vi "Calc Texel Starting Conditions.vi"(10 "Texture":T5, 11 "Sorted Triangle":T1={"Top Vertex"={"Position"={"x"=0.0, "y"=0.0, "z"=0.0}, "UV"={"u"=0.0, "v"=0.0}, "Colour"=12517256}, "Mid Vertex"={"Position"={"x"=0.0, "y"=0.0, "z"=0.0}, "UV"={"u"=0.0, "v"=0.0}, "Colour"=12517256}, "Bottom Vertex"={"Position"={"x"=0.0, "y"=0.0, "z"=0.0}, "UV"={"u"=0.0, "v"=0.0}, "Colour"=12517256}, "Colour"=0} {"Bottom Vertex"."UV"."v" min=0 max=1 step=0.1; "Bottom Vertex"."UV"."u" min=0 max=1 step=0.1; "Mid Vertex"."UV"."v" min=0 max=1 step=0.1; "Mid Vertex"."UV"."u" min=0 max=1 step=0.1; "Top Vertex"."UV"."v" min=0 max=1 step=0.1; "Top Vertex"."UV"."u" min=0 max=1 step=0.1}) -> (3 "Step Deltas (Texels Per Step)":T7)   [LabVIEW 2020]
uses:
  Texel Step Deltas.ctl
  Raster (FPGA).lvlib
  Point 2D (SGL).ctl
  UV.ctl
  Rectangle Dimensions.ctl
  Texture.ctl
  Vector 3D.ctl
  Vertex.ctl
  Triangle (Sorted).ctl
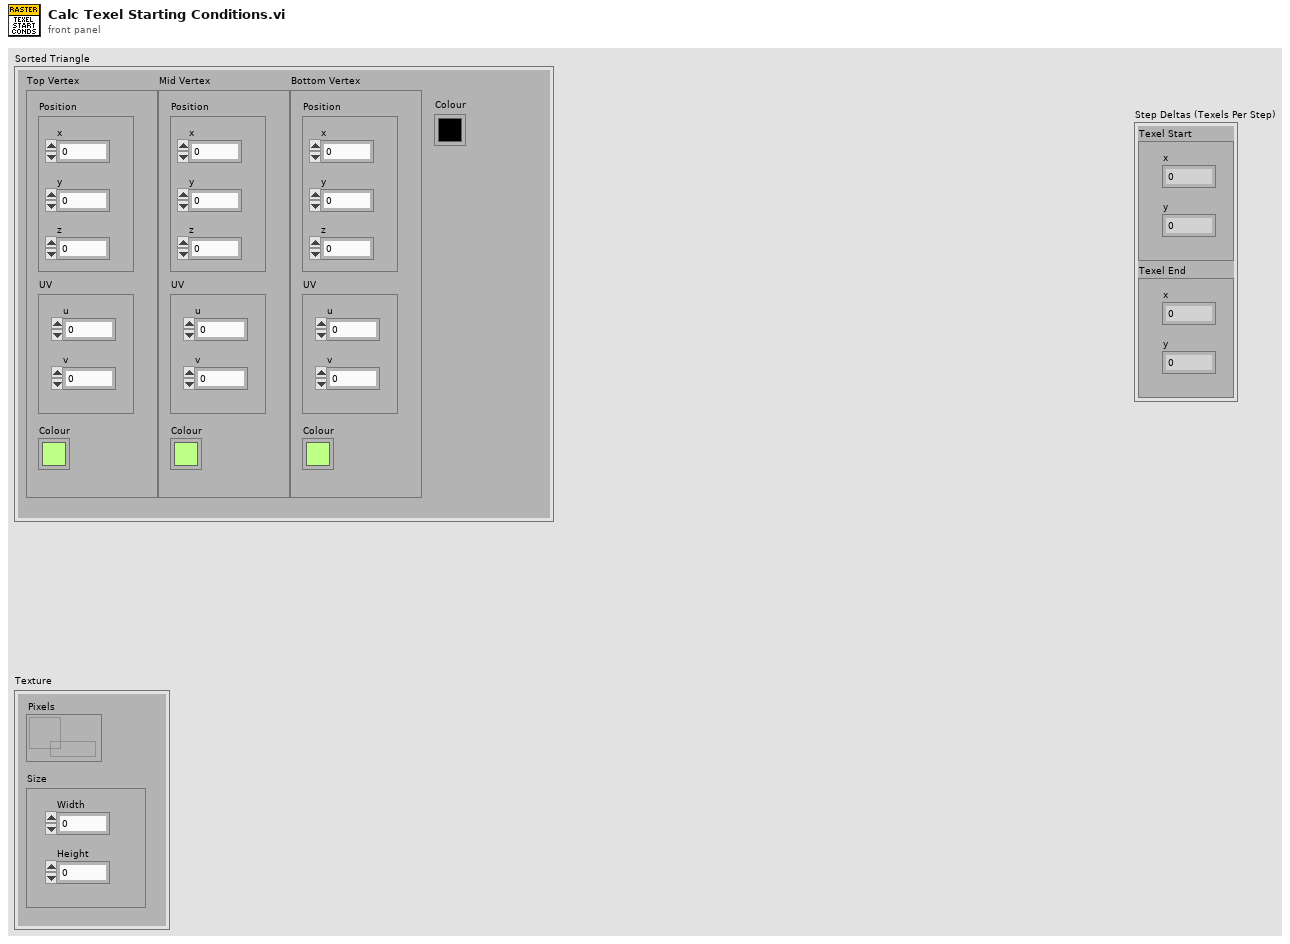
[diagram p1: front panel]
types:
  T1 = typedef "Raster (FPGA).lvlib/Triangle (Sorted).ctl" = cluster{"Top Vertex":T2, "Mid Vertex":T2, "Bottom Vertex":T2, "Colour":u32}
  T2 = typedef "Raster (FPGA).lvlib/Vertex.ctl" = cluster{"Position":T3, "UV":T4, "Colour":u32}
  T3 = typedef "Raster (FPGA).lvlib/Vector 3D.ctl" = cluster{"x":sgl, "y":sgl, "z":sgl}
  T4 = typedef "Raster (FPGA).lvlib/UV.ctl" = cluster{"u":sgl, "v":sgl}
  T5 = typedef "Raster (FPGA).lvlib/Texture.ctl" = cluster{"Pixels":refnum<data-value>, "Size":T6}
  T6 = typedef "Raster (FPGA).lvlib/Rectangle Dimensions.ctl" = cluster{"Width":u32, "Height":u32}
  T7 = typedef "Raster (FPGA).lvlib/Texel Step Deltas.ctl" = cluster{"Texel Start":T8, "Texel End":T8}
  T8 = typedef "Raster (FPGA).lvlib/Point 2D (SGL).ctl" = cluster{"x":sgl, "y":sgl}
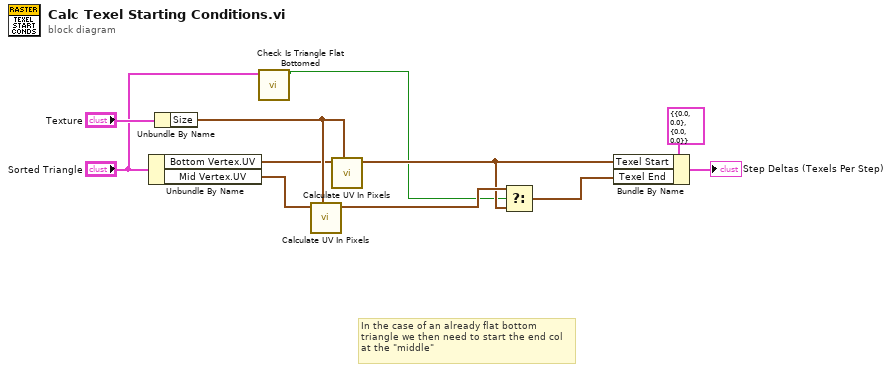
[diagram p0: block diagram]
diagram:
  # "In the case of an already flat bottom triangle we then need to start the end col at the \"middle\""
  n1 = Unbundle By Name("Sorted Triangle") -> ("Bottom Vertex.UV"=w4:T4, "Mid Vertex.UV"=w3:T4)
  n2 = Unbundle By Name("Texture") -> ("Size"=w5:T6)
  n3 = call "Check Is Triangle Flat Bottomed.vi"("Sorted Triangle"="Sorted Triangle") -> ("Flat Bottom Triangle"=w1:bool)  [unwired: 10 in]
  n4 = call "Calculate UV In Pixels.vi"("Texture Dimensions"=w5, "UV"=w3) -> ("Pixels"=w8:T8)  [unwired: 9 in]
  n5 = call "Calculate UV In Pixels.vi"("Texture Dimensions"=w5, "UV"=w4) -> ("Pixels"=w7:T8)  [unwired: 9 in]
  n6 = Select(t=w8, s=w1, f=w7) -> (s? t:f=w11:T8)
  n7 = Bundle By Name(cluster=T7 {"Texel Start"={"x"=0.0, "y"=0.0}, "Texel End"={"x"=0.0, "y"=0.0}} ("Step Deltas (Texels Per Step)"), "Texel Start"=w7, "Texel End"=w11) -> (→"Step Deltas (Texels Per Step)":T7)
